vi "Result.vi"(8 "error in (no error)":errorcluster, 11 "Data2D in":refnum<class "Data2D.lvclass">) -> (0 "error out":errorcluster, 3 "Data2D out":refnum<class "Data2D.lvclass">)   [LabVIEW 2018, in "Data2D.lvclass"]
uses:
  Data2D.lvclass
  Data2D.lvclass/Data2D.ctl
  <vilib>/Utility/file.llb/Write Delimited Spreadsheet (DBL).vi
panel:
  in  "path":path
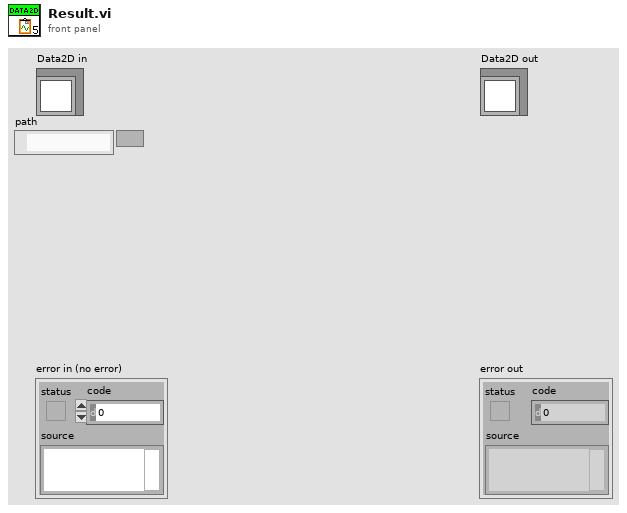
[diagram p1: front panel]
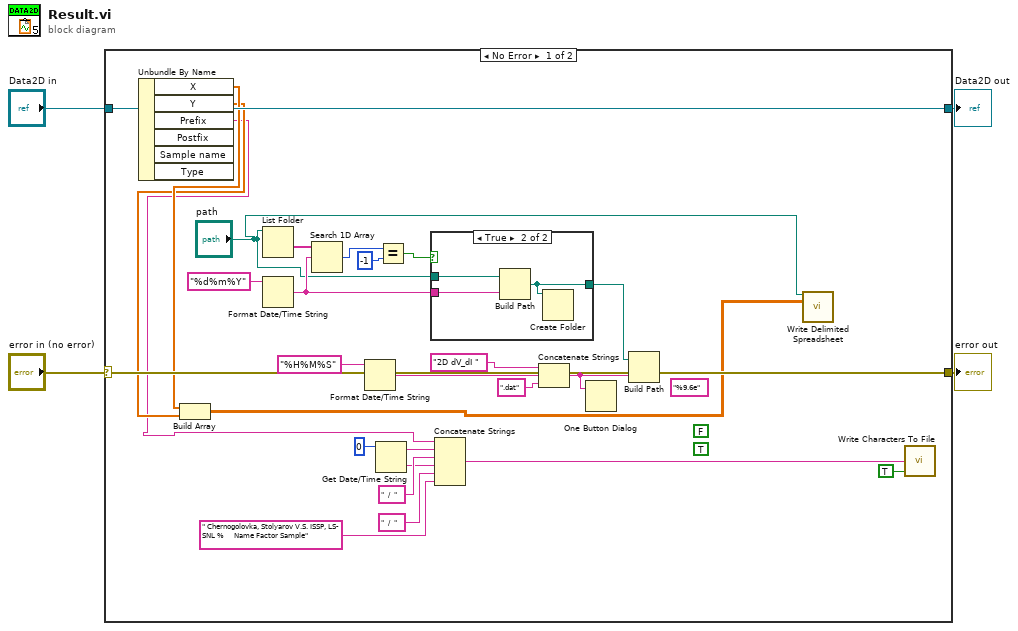
[diagram p0: block diagram]
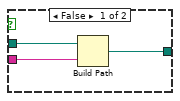
[diagram p2: hidden frame]
diagram:
  n1 = case shown="No Error" "error in (no error)" {
    selector: "error in (no error)" -> [w31 w39]
    tunnel: [w31 w39] -> w3
    tunnel: [w30 w38] -> w1
    tunnel: "Data2D in" -> [w30 w38]
    frame No Error {
      (unwired) TRUE ("transpose? (no:F)")
      (unwired) FALSE ("append to file? (new file:F)")
      (unwired) "%9.6e" ("format (%.3f)")
      n2 = Unbundle By Name(w30) -> ("X"=w9:dbl[], "Y"=w8:dbl[], "Prefix"=w7:string)  [unwired: 3 out]
      n3 = Build Array(w9, w8) -> (w6:dbl[][])
      n4 = List Folder(path="path") -> (folder names=w26:string[])  [unwired: 3 in, 3 out]
      n5 = Format Date/Time String(time format string (%c)="%d%m%Y") -> (date/time string=w10:string)  [unwired: 2 in]
      n6 = Search 1D Array(1D array=w26, element=w10) -> (index of element=w27:i32)  [unwired: 1 in]
      n7 = Format Date/Time String(time format string (%c)="%H%M%S") -> (date/time string=w13:string)  [unwired: 2 in]
      n8 = Get Date/Time String(date format (0)=0) -> (date string=w21:string, time string=w22:string)  [unwired: 2 in]
      n9 = Equal?(x=w27, y=-1) -> (x = y?=w29:bool)
      n10 = case shown="True" w29 {
        tunnel: w10 -> [w34 w37]
        tunnel: [w33 w36] -> w17
        tunnel: "path" -> [w32 w35]
        frame False {
          n11 = Build Path(base path=w32, name or relative path=w34) -> (appended path=w33:path)
        }
        frame True {
          n12 = Build Path(base path=w35, name or relative path=w37) -> (appended path=w36:path)
          n13 = Create Folder(path (use dialog)=w36) -> ()  [unwired: 2 in, 3 out]
        }
      }
      n14 = Concatenate Strings(w7, w21, "  /  " ("date string"), w22, "  /  " ("date string"), " Chernogolovka, Stolyarov V.S. ISSP, LS- SNL %     Name Factor Sample" ("date string")) -> (w20:string)
      n15 = Concatenate Strings("2D dV_dI " ("string"), w13, ".dat" ("substring")) -> (w16:string)
      n16 = One Button Dialog(message=w16) -> ()  [unwired: 1 in, 1 out]
      n17 = Build Path(base path=w17, name or relative path=w16) -> ()  [unwired: 1 out]
      n18 = call-poly <vilib>:"Write Delimited Spreadsheet.vi"("file path (dialog if empty)"="path", "2D data"=w6) -> ()  [unwired: 12 in, 2 out]
      n19 = call <vilib>:"Write Characters To File.vi"("append to file? (new file:F)"=TRUE, "character string"=w20) -> ()  [unwired: 3 in, 1 out]
    }
    frame Error {
    }
  }
  "error out" <- w3
  "Data2D out" <- w1
